vi "chaosui-crest-cu-setstate.vi"(5 "dev_state":T1=enum."init", 6 "timeout (10000)":i32=10000, 7 "cuname":string, 8 "handleConnection":T3) -> (0 "dev_error":bool, 1 "timestamp":u64, 2 "nok":i32, 3 "dev_state_out":T1, 4 "output out":string)   [LabVIEW 2012]
doc: "uint64_t chaos_crest_cu_get(chaos_crest_handle_t h,const char*cuname,char*output,int maxsize);"
uses:
  chaosui-crest.lvlib
  <vilib>/httpClient/ClientHandle.ctl
  <vilib>/httpClient/LabVIEWHTTPClient.lvlib
  ChaosDevState.ctl
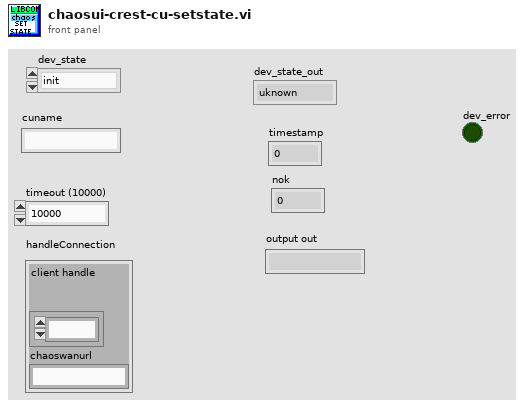
[diagram p1: front panel]
types:
  T1 = typedef "ChaosDevState.ctl" = enum16{"uknown", "stop", "init", "deinit", "start"}
  T2 = typedef "LabVIEWHTTPClient.lvlib/ClientHandle.ctl" = refnum<k1>
  T3 = cluster{"client handle":T2, "chaoswanurl":string}
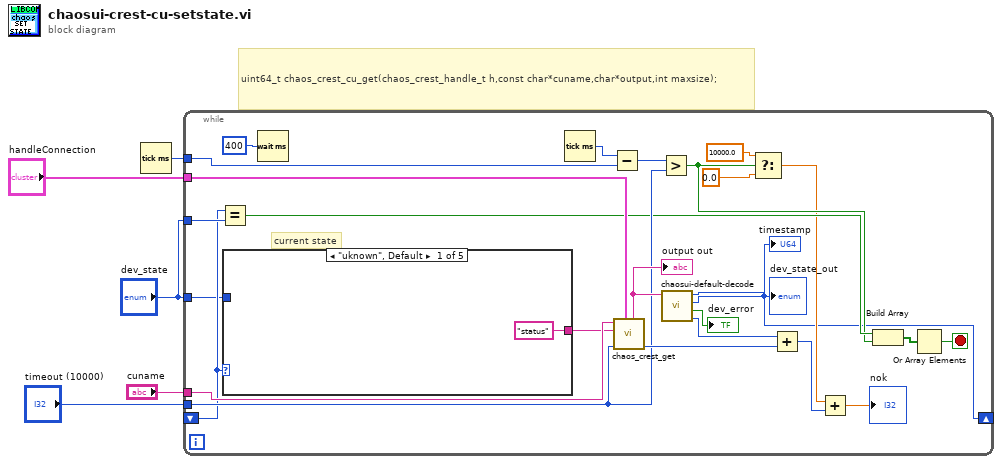
[diagram p0: block diagram]
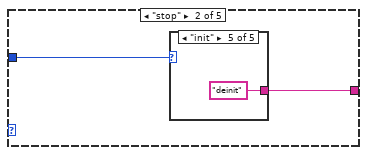
[diagram p2: hidden frame]
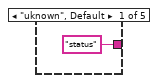
[diagram p3: hidden frame]
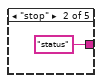
[diagram p4: hidden frame]
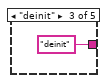
[diagram p5: hidden frame]
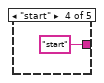
[diagram p6: hidden frame]
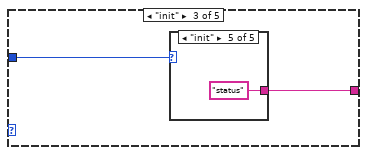
[diagram p7: hidden frame]
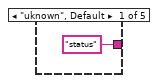
[diagram p8: hidden frame]
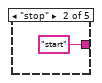
[diagram p9: hidden frame]
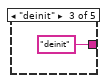
[diagram p10: hidden frame]
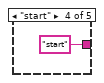
[diagram p11: hidden frame]
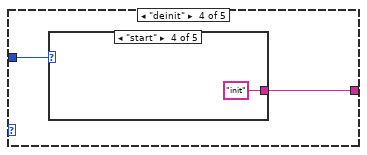
[diagram p12: hidden frame]
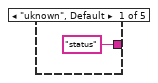
[diagram p13: hidden frame]
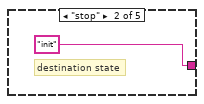
[diagram p14: hidden frame]
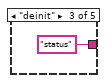
[diagram p15: hidden frame]
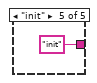
[diagram p16: hidden frame]
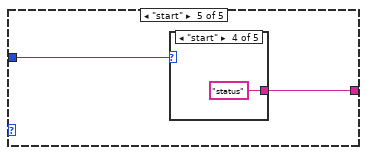
[diagram p17: hidden frame]
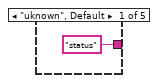
[diagram p18: hidden frame]
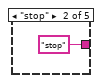
[diagram p19: hidden frame]
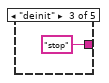
[diagram p20: hidden frame]
diagram:
  # "uint64_t chaos_crest_cu_get(chaos_crest_handle_t h,const char*cuname,char*output,int maxsize);"
  n1 = Tick Count (ms)() -> (millisecond timer value=w2:u32)
  n2 = while {
    tunnel: "handleConnection" -> [w28]
    tunnel: "timeout (10000)" -> [w19]
    tunnel: "cuname" -> [w27]
    tunnel: "dev_state" -> [w10]
    tunnel: w2 -> [w20]
    shift-right: [w8] -> _
    shift-left: _ -> [w7]
    tunnel: "dev_state" -> [w6]
    stop <- w24 stop-if-true
    # "current state"
    n3 = Equal?(x=w7, y=w10) -> (x = y?=w17:bool)
    n4 = case shown="\"uknown\", Default" w7 {
      tunnel: ["status" w33 w40 w47 w54] -> w9
      tunnel: w6 -> [_ w34 w41 w48 w55]
      frame "uknown", Default {
      }
      frame "stop" {
        n5 = case shown="\"init\"" w34 {
          tunnel: ["status" "status" "deinit" "start" "deinit"] -> w33
          frame "uknown", Default {
          }
          frame "stop" {
          }
          frame "deinit" {
          }
          frame "start" {
          }
          frame "init" {
          }
        }
      }
      frame "init" {
        n6 = case shown="\"init\"" w41 {
          tunnel: ["status" "start" "deinit" "start" "status"] -> w40
          frame "uknown", Default {
          }
          frame "stop" {
          }
          frame "deinit" {
          }
          frame "start" {
          }
          frame "init" {
          }
        }
      }
      frame "deinit" {
        n7 = case shown="\"start\"" w48 {
          tunnel: ["status" "init" "status" "init" "init"] -> w47
          frame "uknown", Default {
          }
          frame "stop" {
            # "destination state"
          }
          frame "deinit" {
          }
          frame "start" {
          }
          frame "init" {
          }
        }
      }
      frame "start" {
        n8 = case shown="\"start\"" w55 {
          tunnel: ["status" "stop" "stop" "status" "stop"] -> w54
          frame "uknown", Default {
          }
          frame "stop" {
          }
          frame "deinit" {
          }
          frame "start" {
          }
          frame "init" {
          }
        }
      }
    }
    n9 = Wait (ms)(milliseconds to wait=u32 400) -> ()  [unwired: 1 out]
    n10 = Tick Count (ms)() -> (millisecond timer value=w21:u32)
    n11 = Subtract(x=w21, y=w20) -> (x-y=w18:u32)
    n12 = call "chaos_crest_get.vi"("cuname"=w27, "cmd"=w9, "timeout (10000)"=w19, "handleConnection"=w28) -> ("body"=w26:string, "nok"=w25:i32)  [unwired: 4 in, 1 out]
    "output out" <- w26
    n13 = Greater?(x=w18, y=w19) -> (0:w14:bool)
    n14 = call "chaosui-default-decode.vi"("JSON string"=w26) -> ("parse_error"=w29:i32, "dev_error"=→"dev_error":bool, "dev_state"=w8:T1, "timestamp"=→"timestamp":u64)  [unwired: 3 in, 1 out]
    "dev_state_out" <- w8
    n15 = Select(t=10000.0, s=w14, f=0.0) -> (s? t:f=w11:dbl)
    n16 = Add(x=w29, y=w25) -> (x+y=w23:i32)
    n17 = Add(x=w11, y=w23) -> (x+y=→"nok":dbl)
    n18 = Build Array(w17, w14) -> (w16:bool[])
    n19 = Or Array Elements(Boolean array=w16) -> (logical OR=w24:bool)
  }
